vi "switch.vi"() -> ()   [LabVIEW 2017]
panel:
  out "Time":dbl caption="Elapsed Time (s)"
  out "LED":bool
  in  "SWITCH 2":bool
  out "Time":dbl caption="Elapsed Time (s)"
  out "LED":bool
  in  "SWITCH":bool
  out "Time":dbl caption="Elapsed Time (s)"
  out "LED":bool
  in  "SWITCH":bool
  in  "?":bool
  out "Time":dbl caption="Elapsed Time (s)"
  out "LED":bool
  in  "SWITCH":bool
  out "Time":dbl caption="Elapsed Time (s)"
  in  "SWITCH":bool
  out "LED":bool
  out "TIME":dbl caption="Elapsed Time (s)"
  out "LED 2":bool
  in  "SWITCH":bool
  # "SWITCH WHEN PRESSED"
  # "SWITCH WHEN RELEASED"
  # "LATCH WHEN PRESSED"
  # "SWITCH UNTILL RELEASED"
  # "LATCH WHEN RELEASED"
  # "LATCH UNTIL RELEASED"
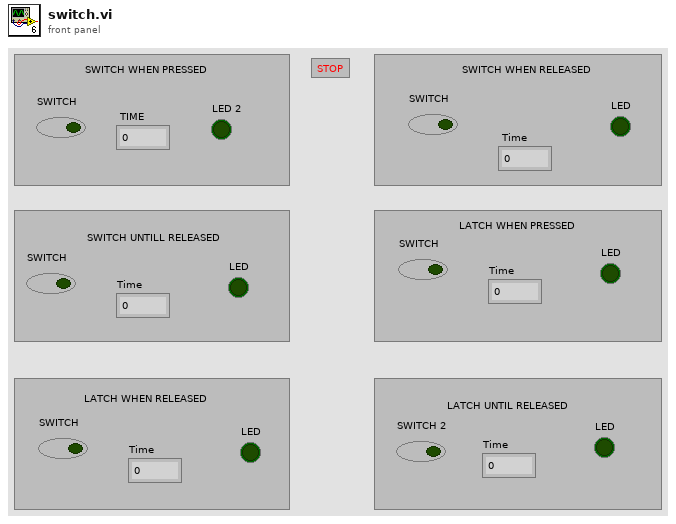
[diagram p1: front panel]
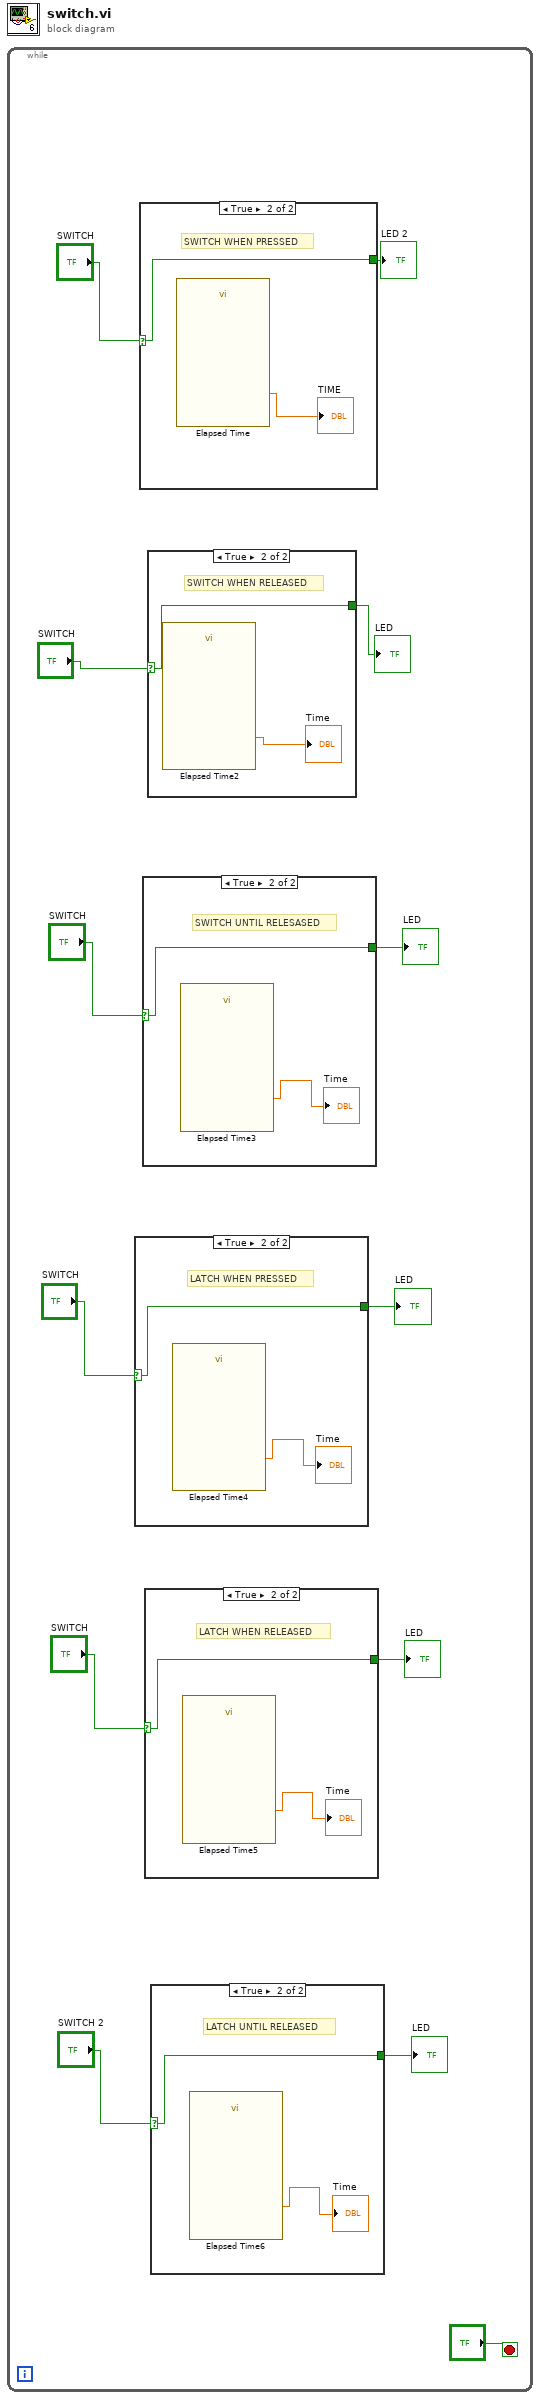
[diagram p0: block diagram]
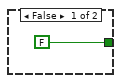
[diagram p2: hidden frame]
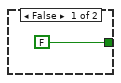
[diagram p3: hidden frame]
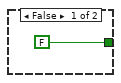
[diagram p4: hidden frame]
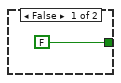
[diagram p5: hidden frame]
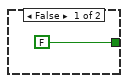
[diagram p6: hidden frame]
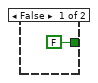
[diagram p7: hidden frame]
diagram:
  n1 = while {
    stop <- "?" stop-if-true
    n2 = case shown="True" "SWITCH" {
      selector: "SWITCH" -> [_ w22]
      tunnel: [FALSE w22] -> w5
      frame False {
      }
      frame True {
        # "LATCH WHEN PRESSED"
        n3 = call "Elapsed Time4"() -> ("Elapsed Time (s)"=→"Time":dbl)  [unwired: 12 in, 7 out]
      }
    }
    "LED" <- w5
    n4 = case shown="True" "SWITCH" {
      selector: "SWITCH" -> [_ w31]
      tunnel: [FALSE w31] -> w12
      frame False {
      }
      frame True {
        # "SWITCH WHEN PRESSED"
        n5 = call "Elapsed Time"() -> ("Elapsed Time (s)"=→"TIME":dbl)  [unwired: 12 in, 7 out]
      }
    }
    "LED 2" <- w12
    n6 = case shown="True" "SWITCH" {
      selector: "SWITCH" -> [_ w25]
      tunnel: [FALSE w25] -> w8
      frame False {
      }
      frame True {
        # "SWITCH UNTIL RELESASED"
        n7 = call "Elapsed Time3"() -> ("Elapsed Time (s)"=→"Time":dbl)  [unwired: 12 in, 7 out]
      }
    }
    "LED" <- w8
    n8 = case shown="True" "SWITCH" {
      selector: "SWITCH" -> [_ w19]
      tunnel: [FALSE w19] -> w3
      frame False {
      }
      frame True {
        # "LATCH WHEN RELEASED"
        n9 = call "Elapsed Time5"() -> ("Elapsed Time (s)"=→"Time":dbl)  [unwired: 12 in, 7 out]
      }
    }
    "LED" <- w3
    n10 = case shown="True" "SWITCH" {
      selector: "SWITCH" -> [_ w28]
      tunnel: [FALSE w28] -> w10
      frame False {
      }
      frame True {
        # "SWITCH WHEN RELEASED"
        n11 = call "Elapsed Time2"() -> ("Elapsed Time (s)"=→"Time":dbl)  [unwired: 12 in, 7 out]
      }
    }
    "LED" <- w10
    n12 = case shown="True" "SWITCH 2" {
      selector: "SWITCH 2" -> [_ w16]
      tunnel: [FALSE w16] -> w1
      frame False {
      }
      frame True {
        # "LATCH UNTIL RELEASED"
        n13 = call "Elapsed Time6"() -> ("Elapsed Time (s)"=→"Time":dbl)  [unwired: 12 in, 7 out]
      }
    }
    "LED" <- w1
  }
